vi "Laboratory_practice5.vi"() -> ()   [LabVIEW 2014]
panel:
  in  "stop":bool
  out "RMS":dbl
  out "Waveform Graph":dynamicdata(graph)
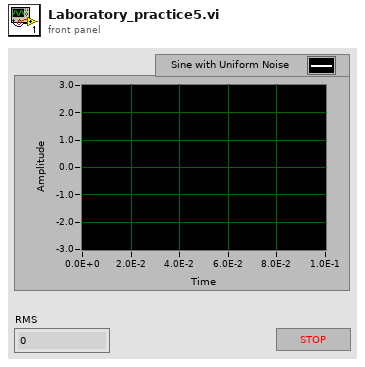
[diagram p1: front panel]
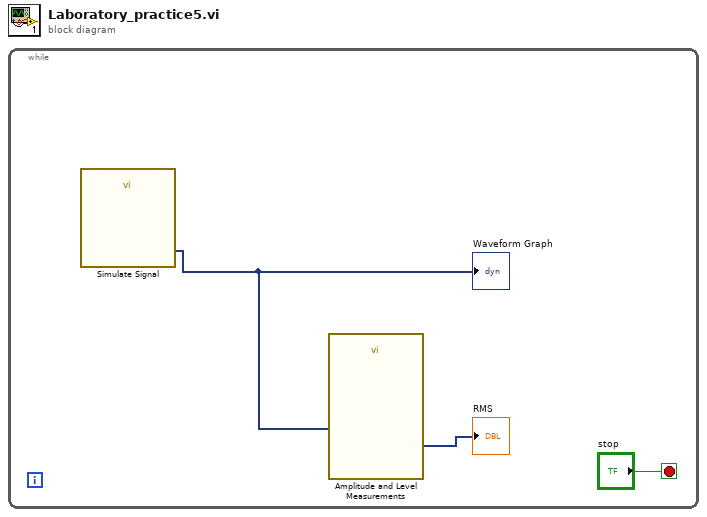
[diagram p0: block diagram]
diagram:
  n1 = while {
    stop <- "stop" stop-if-true
    n2 = call "Simulate Signal"() -> ("Sine"=w1:dynamicdata)  [unwired: 14 in, 1 out]
    "Waveform Graph" <- w1
    n3 = call "Amplitude and Level Measurements"("Signals"=w1) -> ("RMS"=→"RMS":dynamicdata)  [unwired: 12 in, 2 out]
  }
